vi "Set Alternating BD Colours.vi"(8 "error in (no error)":errorcluster) -> (0 "error out":errorcluster)   [LabVIEW 2020]
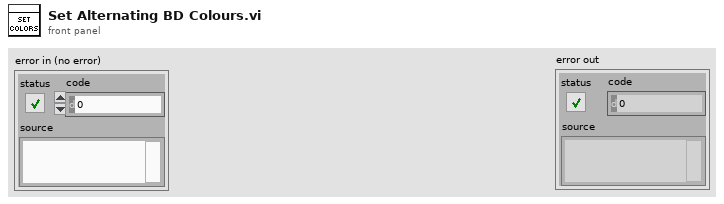
[diagram p1: front panel]
types:
  T1 = enum32{"Invalid", "Standard", "Closed", "Hidden", "Minimized", "Maximized"}
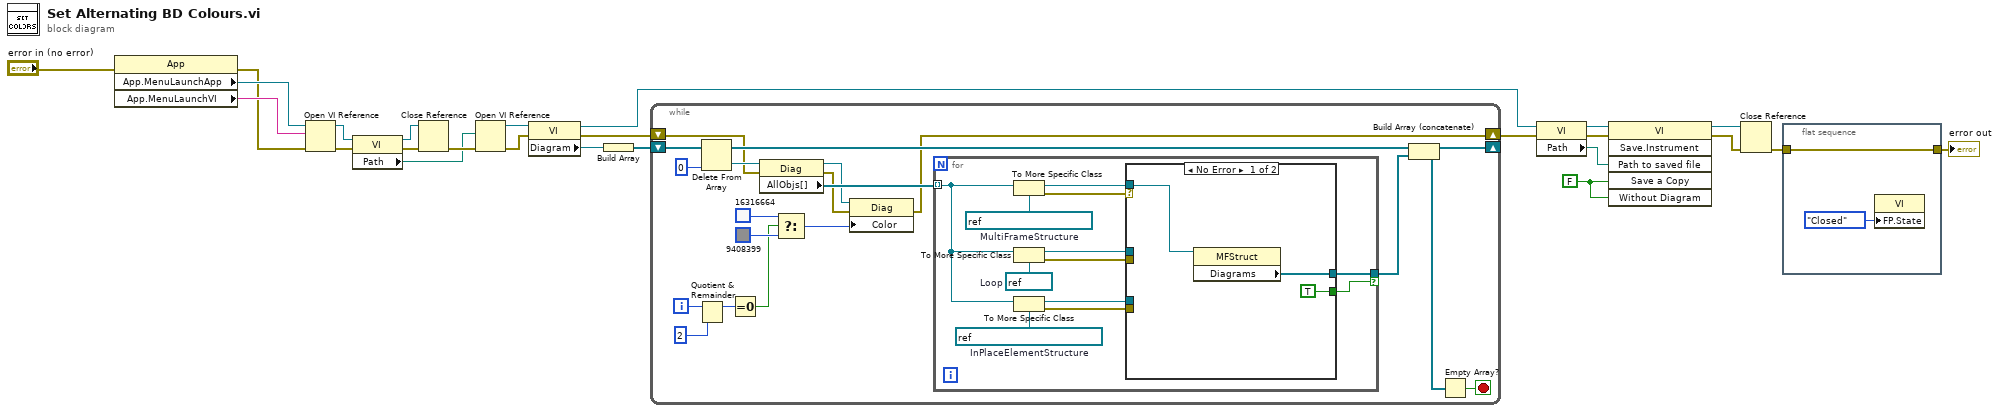
[diagram p0: block diagram]
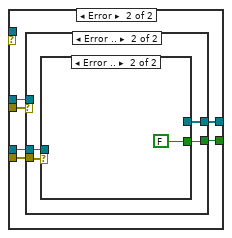
[diagram p2: hidden frame]
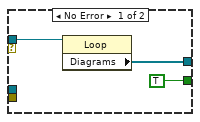
[diagram p3: hidden frame]
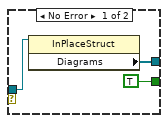
[diagram p4: hidden frame]
diagram:
  w17 = FALSE
  n1 = property class="App"(error in="error in (no error)") -> (error out=w12:errorcluster, "App.MenuLaunchApp"=w13:refnum<vi>, "App.MenuLaunchVI"=w14:string)  [unwired: 1 in, 1 out]
  n2 = Open VI Reference(application reference (local)=w13, vi path=w14, error in (no error)=w12) -> (vi reference=w10:refnum<vi>, error out=w9:errorcluster)  [unwired: 3 in]
  n3 = property class="VI"(reference=w10, error in=w9) -> (reference out=w8:refnum<vi>, error out=w7:errorcluster, "Path"=w3:path)
  n4 = Close Reference(reference=w8, error in (no error)=w7) -> (error out=w4:errorcluster)
  n5 = Open VI Reference(vi path=w3, error in (no error)=w4) -> (vi reference=w6:refnum<vi>, error out=w5:errorcluster)  [unwired: 4 in]
  n6 = property class="VI"(reference=w6, error in=w5) -> (reference out=w21:refnum<vi>, error out=w23:errorcluster, "Diagram"=w25:refnum<vi>)
  n7 = Build Array(w25) -> (w24:refnum<vi>[])
  n8 = while {
    shift-right: [w37] -> _
    shift-left: w24 -> [w44]
    shift-right: [w26] -> w22
    shift-left: w23 -> [w28]
    i -> [w36]
    stop <- w38 stop-if-true
    n9 = Quotient & Remainder(x=w36, y=2) -> (x-y*floor(x/y)=w32:i32)  [unwired: 1 out]
    n10 = Delete From Array(array=w44, index=0) -> (deleted portion=w42:refnum<vi>, array with subset deleted=w40:refnum<vi>[])  [unwired: 1 in]
    n11 = Equal To 0?(x=w32) -> (x = 0?=w31:bool)
    n12 = property class="Diag"(reference=w42, error in=w28) -> (reference out=w30:refnum<vi>, error out=w27:errorcluster, "AllObjs[]"=w41:refnum<vi>[])
    n13 = Select(t=u32 16316664, s=w31, f=u32 9408399) -> (s? t:f=w29:u32)
    n14 = property class="Diag"(reference=w30, error in=w27, "Color"=w29) -> (error out=w26:errorcluster)  [unwired: 1 out]
    n15 = for {
      tunnel: w41 -> [w53] mode=indexing
      tunnel: [w46] -> w39 if=w45
      w54 = refnum<vi> refnum  # InPlaceElementStructure
      w55 = refnum<vi> refnum  # Loop
      w56 = refnum<vi> refnum  # MultiFrameStructure
      n16 = To More Specific Class(target class=w56, reference=w53) -> (specific class reference=w51:refnum<vi>, error out=w52:errorcluster)  [unwired: 1 in]
      n17 = To More Specific Class(target class=w55, reference=w53) -> (specific class reference=w49:refnum<vi>, error out=w50:errorcluster)  [unwired: 1 in]
      n18 = To More Specific Class(target class=w54, reference=w53) -> (specific class reference=w47:refnum<vi>, error out=w48:errorcluster)  [unwired: 1 in]
      n19 = case shown="No Error" w52 {
        tunnel: w51 -> [w59 _]
        tunnel: w50 -> [_ w65]
        tunnel: w49 -> [_ w64]
        tunnel: w48 -> [_ w61]
        tunnel: w47 -> [_ w60]
        tunnel: [w58 w63] -> w46
        tunnel: [TRUE w62] -> w45
        frame No Error {
          n20 = property class="MFStruct"(reference=w59) -> ("Diagrams"=w58:refnum<vi>[])  [unwired: 1 in, 2 out]
        }
        frame Error {
          n21 = case shown="Error .." w65 {
            tunnel: w64 -> [w68 _]
            tunnel: [w67 w70] -> w63
            tunnel: [TRUE w69] -> w62
            tunnel: w61 -> [_ w72]
            tunnel: w60 -> [_ w71]
            frame No Error {
              n22 = property class="Loop"(reference=w68) -> ("Diagrams"=w67:refnum<vi>[])  [unwired: 1 in, 2 out]
            }
            frame Error {
              n23 = case shown="Error .." w72 {
                tunnel: w71 -> [w75 _]
                tunnel: [w74 _] -> w70
                tunnel: [TRUE FALSE] -> w69
                frame No Error {
                  n24 = property class="InPlaceStruct"(reference=w75) -> ("Diagrams"=w74:refnum<vi>[])  [unwired: 1 in, 2 out]
                }
                frame Error {
                }
              }
            }
          }
        }
      }
    }
    n25 = Build Array (concatenate)(w40, w39) -> (w37:refnum<vi>[])
    n26 = Empty Array?(array=w37) -> (empty?=w38:bool)
  }
  n27 = property class="VI"(reference=w21, error in=w22) -> (reference out=w19:refnum<vi>, error out=w20:errorcluster, "Path"=w18:path)
  n28 = invoke class="VI" method="Save.Instrument"(reference=w19, error in=w20, "Path to saved file"=w18, "Save a Copy"=w17, "Without Diagram"=w17) -> (reference out=w16:refnum<vi>, error out=w15:errorcluster)  [unwired: 1 in, 4 out]
  n29 = Close Reference(reference=w16, error in (no error)=w15) -> (error out=w1:errorcluster)
  n30 = flat-sequence {
    tunnel: [w78] -> w2
    tunnel: w1 -> [w78]
    frame #0 {
      n31 = property class="VI"("FP.State"=T1."Closed" ("Front Panel Window:State")) -> ()  [unwired: 2 in, 2 out]
    }
  }
  "error out" <- w2
